vi "CountPrimes.vi"(8 "error in (no error)":errorcluster, 11 "Prime_Sieve in":refnum<class "Prime_Sieve.lvclass">) -> (0 "error out":errorcluster, 2 "Count":i32, 3 "Prime_Sieve out":refnum<class "Prime_Sieve.lvclass">)   [LabVIEW 2020, in "Prime_Sieve.lvclass"]
uses:
  Prime_Sieve.lvclass
  Prime_Sieve.lvclass/Prime_Sieve.ctl
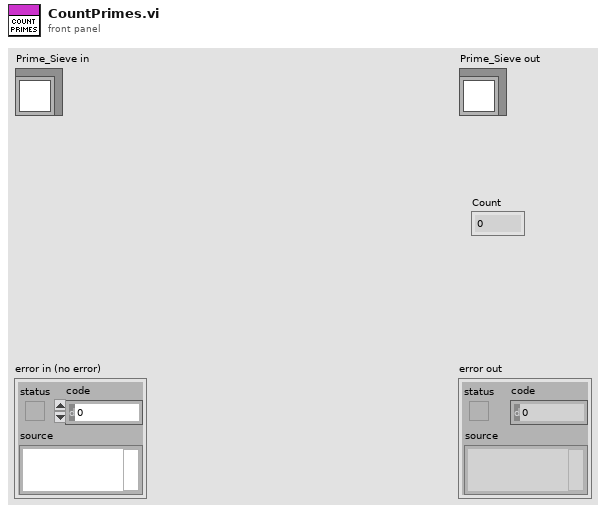
[diagram p1: front panel]
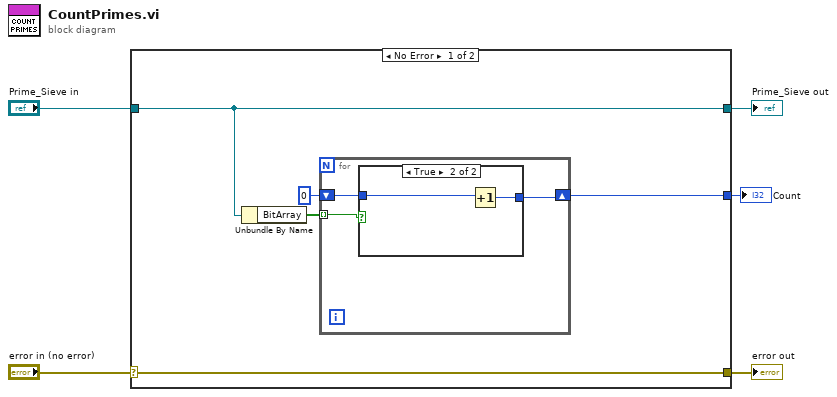
[diagram p0: block diagram]
diagram:
  n1 = case shown="No Error" "error in (no error)" {
    selector: "error in (no error)" -> [w10 w18]
    tunnel: [w10 w18] -> w4
    tunnel: [w9 w17] -> w2
    tunnel: "Prime_Sieve in" -> [w9 w17]
    tunnel: [w6 _] -> w1
    frame No Error {
      n2 = Unbundle By Name(w9) -> ("BitArray"=w8:bool[])
      n3 = for {
        tunnel: w8 -> [w13] mode=indexing
        shift-right: [w11] -> w6
        shift-left: 0 -> [w12]
        n4 = case shown="True" w13 {
          tunnel: w12 -> [w14 w16]
          tunnel: [w14 w15] -> w11
          frame False {
          }
          frame True {
            n5 = Increment(x=w16) -> (x+1=w15:i32)
          }
        }
      }
    }
    frame Error {
    }
  }
  "error out" <- w4
  "Prime_Sieve out" <- w2
  "Count" <- w1
